vi "ExDriver.vi"(4 "Error In":errorcluster, 7 "Command":string) -> (0 "Error Out":errorcluster, 3 "Response":string)   [LabVIEW 2018]
uses:
  MOKO_LabViewLibrary/MokoLowLevel/MokoLowLovelControl/MLLC_DriverName.ctl
  MOKO_LabViewLibrary/MokoLowLevel/MokoLowLovelControl/MLLC_ConnectCluster.ctl
  MOKO_LabViewLibrary/MokoLowLevel/MokoLowLovelControl/MLLC_InterfaceType.ctl
  MOKO_LabViewLibrary/MokoLowLevel/MokoLowLovelControl/MLLC_OpenedSession.ctl
  MOKO_LabViewLibrary/MokoLowLevel/MokoLowLovelControl/MLLC_InterfaceSettings.ctl
  MOKO_LabViewLibrary/MokoLowLevel/MokoLowLovelControl/MLLC_InterfaceKind.ctl
  MOKO_LabViewLibrary/MokoLowLevel/MokoLowLovelControl/MLLC_Request.ctl
  MOKO_LabViewLibrary/MokoLowLevel/MokoLowLovelControl/MLLC_ResponseInit.ctl
panel:
  in  "Response Init":T1="43B"
  in  "Request":T2="ID"
  in  "Settings":T8={"Saved Data"=variant, "Permanent data"={"Connect"={"InterfaceType"=enum."VISA", "OpenedSession"="", "InterfaceSettings"={"Interface"=enum."RS232", "EOS 4 read"=enum."LF (\\n)", "EOS 4 write"=enum."LF (\\n)", "TMO, ms"=10000, "Sett"=variant(cluster{"Baud Rate":u32, "Data Bits":u16, "Parity":u16, "Stop Bits":u16, "Flow Control":u16, "Eho":bool} {"Baud Rate"=75, "Data Bits"=0, "Parity"=0, "Stop Bits"=0, "Flow Control"=0, "Eho"=FALSE})}}, "Values"={"Value"=0.0}}}
  in  "Error Code":u32
  in  "Driver Name":T9="ExDriver"
  in  "Mode":T10(ring)
  # "ExDriver"
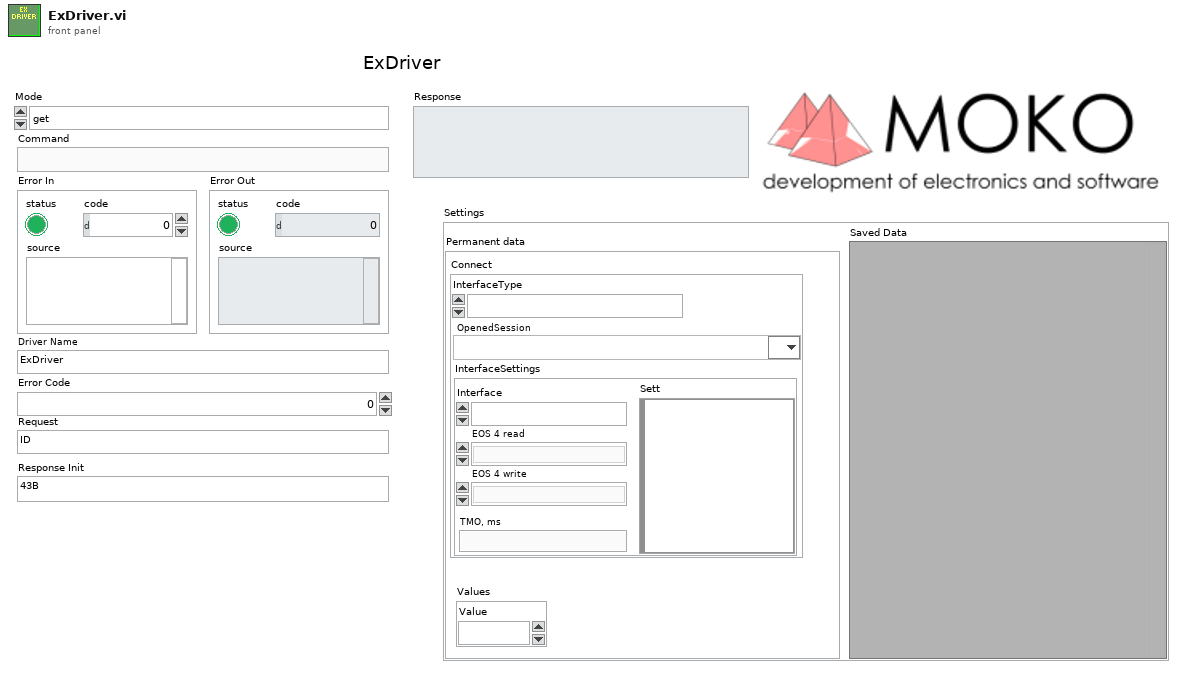
[diagram p1: front panel]
types:
  T1 = typedef "MLLC_ResponseInit.ctl" = string
  T2 = typedef "MLLC_Request.ctl" = string
  T3 = typedef "MLLC_ConnectCluster.ctl" = cluster{"InterfaceType":T4, "OpenedSession":T5, "InterfaceSettings":T6}
  T4 = typedef "MLLC_InterfaceType.ctl" = enum16{"VISA", "Prologix USB-GPIB"}
  T5 = typedef "MLLC_OpenedSession.ctl" = refnum<visa-resource-name>
  T6 = typedef "MLLC_InterfaceSettings.ctl" = cluster{"Interface":T7, "EOS 4 read":enum16{"Default (=EOS 4 write)", "CR (\\r)", "LF (\\n)", "None"}, "EOS 4 write":enum16{"CR+LF (\\r\\n)", "CR (\\r)", "LF (\\n)", "None"}, "TMO, ms":i32, "Sett":variant}
  T7 = typedef "MLLC_InterfaceKind.ctl" = enum16{"RS232", "GPIB", "USB", "Ethernet", "another"}
  T8 = cluster{"Saved Data":variant, "Permanent data":cluster{"Connect":T3, "Values":cluster{"Value":dbl}}}
  T9 = typedef "MLLC_DriverName.ctl" = string
  T10 = enum16{"get", "set", "close", "Init", "Check", "ID"}
  T11 = cluster{"Connect":T3, "Values":cluster{"Value":dbl}}
  T12 = typedef "MLLC_Mode.ctl" = enum16{"get", "set", "close", "Init", "Check"}
  T13 = typedef "MLLC_Error.ctl" = errorcluster
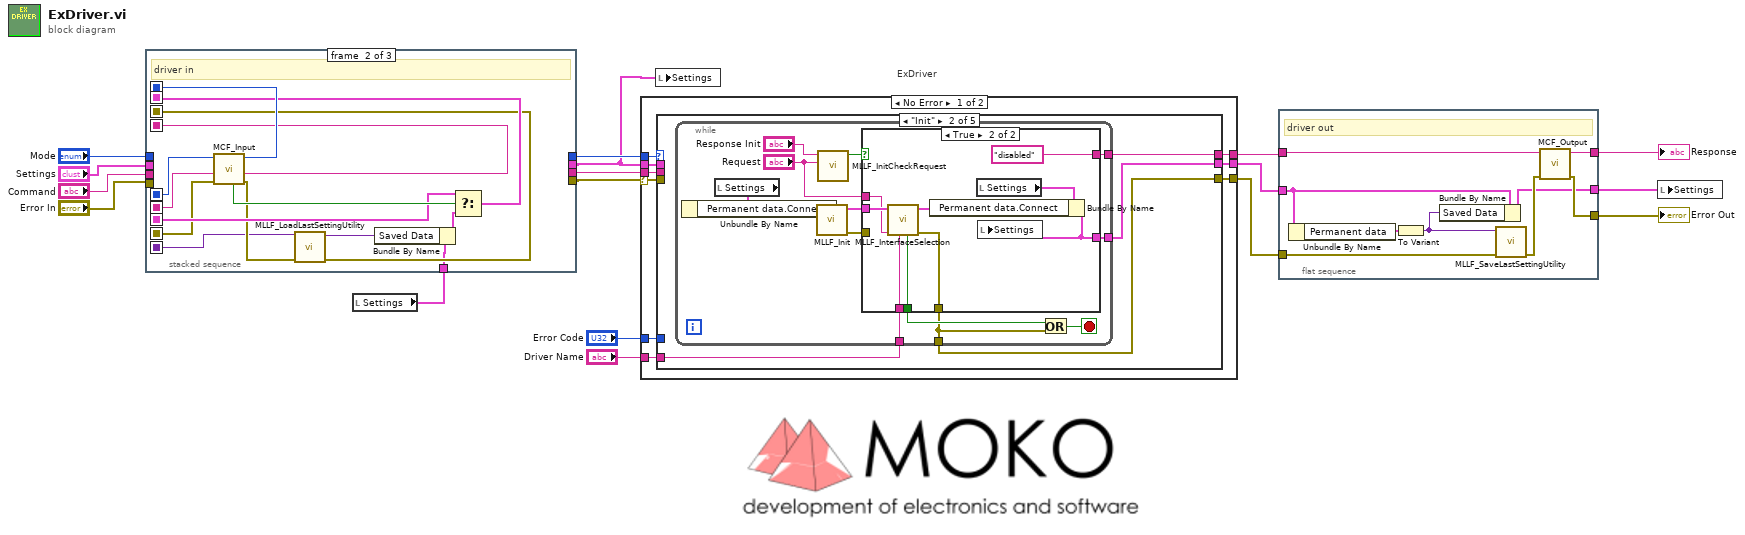
[diagram p0: block diagram]
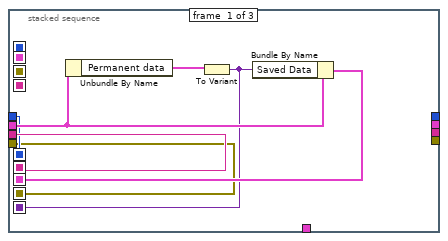
[diagram p2: hidden frame]
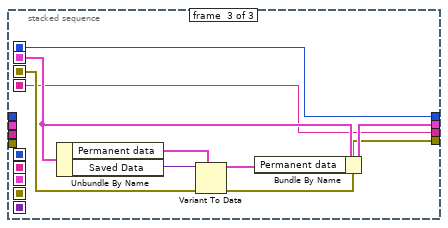
[diagram p3: hidden frame]
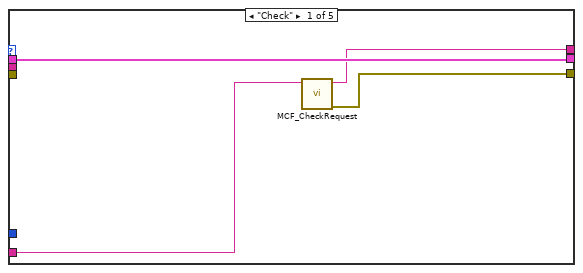
[diagram p4: hidden frame]
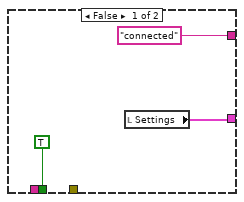
[diagram p5: hidden frame]
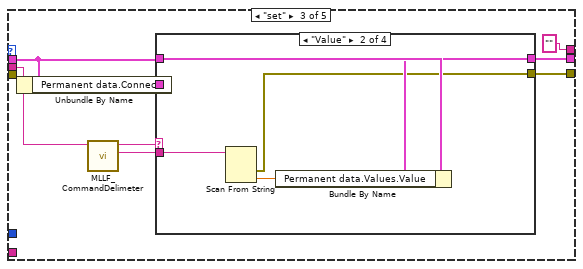
[diagram p6: hidden frame]
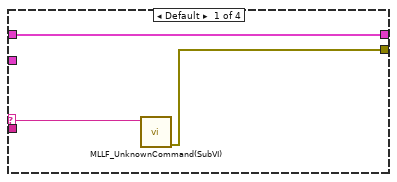
[diagram p7: hidden frame]
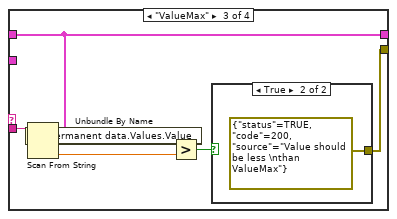
[diagram p8: hidden frame]
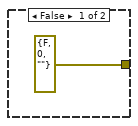
[diagram p9: hidden frame]
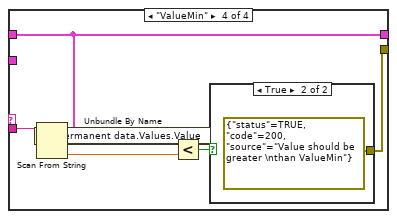
[diagram p10: hidden frame]
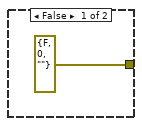
[diagram p11: hidden frame]
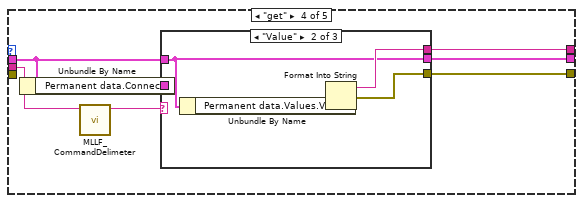
[diagram p12: hidden frame]
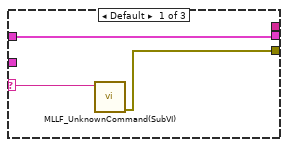
[diagram p13: hidden frame]
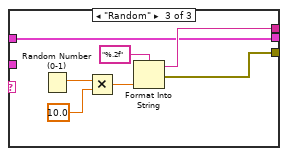
[diagram p14: hidden frame]
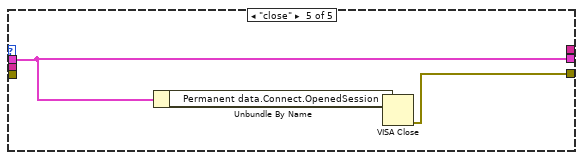
[diagram p15: hidden frame]
diagram:
  # "ExDriver"
  n1 = local read "Settings"() -> (w9:T8)
  n2 = stacked-sequence {
    seq-local: [w20 _ _] -> [_ w36 _]
    seq-local: [w19 _ _] -> [_ w37 _]
    seq-local: [w22 _ _] -> [_ w32 _]
    seq-local: [w18 _ _] -> [_ w31 _]
    seq-local: [w21 _ _] -> [_ w27 _]
    seq-local: [_ w28 _] -> [_ _ w44]
    seq-local: [_ w38 _] -> [_ _ w41]
    seq-local: [_ w35 _] -> [_ _ w40]
    seq-local: [_ w34 _] -> [_ _ w45]
    tunnel: "Command" -> [w20 _ _]
    tunnel: "Mode" -> [w19 _ _]
    tunnel: "Error In" -> [w18 _ _]
    tunnel: "Settings" -> [w23 _ _]
    tunnel: w9 -> [_ w26 _]
    tunnel: [_ _ w40] -> w5
    tunnel: [_ _ w43] -> w6
    tunnel: [_ _ w42] -> w4
    tunnel: [_ _ w41] -> w7
    frame #0 {
      n3 = Unbundle By Name(w23) -> ("Permanent data"=w24:T11)
      n4 = To Variant(anything=w24) -> (Variant=w21:variant)
      n5 = Bundle By Name(cluster=w23, "Saved Data"=w21) -> (w22:T8)
    }
    frame #1 {
      # "driver in"
      n6 = call "MCF_Input.vi"("Error In"=w31, "Command in"=w36, "Mode in"=w37) -> ("Error Out"=w30:errorcluster, "Command out"=w35:string, "Mode out"=w38:T12, "Boolean"=w33:bool)  [unwired: 5 in]
      n7 = call "MLLF_LoadLastSettingUtility.vi"("Error In"=w30, "Save data in"=w27) -> ("Error Out"=w28:errorcluster, "Save data out"=w25:variant)  [unwired: 8 in]
      n8 = Bundle By Name(cluster=w26, "Saved Data"=w25) -> (w29:T8)
      n9 = Select(t=w32, s=w33, f=w29) -> (s? t:f=w34:T8)
    }
    frame #2 {
      n10 = Unbundle By Name(w45) -> ("Permanent data"=w46:T11, "Saved Data"=w39:variant)
      n11 = Variant To Data(error in=w44, type=w46, Variant=w39) -> (data=w47:T11, error out=w42:errorcluster)
      n12 = Bundle By Name(cluster=w45, "Permanent data"=w47) -> (w43:T8)
    }
  }
  n13 = case shown="No Error" w4 {
    selector: w4 -> [w52 w147]
    tunnel: [w54 w147] -> w13
    tunnel: w7 -> [w56 _]
    tunnel: [w55 _] -> w15
    tunnel: w5 -> [w53 _]
    tunnel: w6 -> [w49 w146]
    tunnel: "Error Code" -> [w51 _]
    tunnel: "Driver Name" -> [w50 _]
    tunnel: [w48 w146] -> w14
    frame No Error {
      n14 = case shown="\"Init\"" w56 {
        tunnel: [w58 w62 "" ("Output String") w122 _] -> w55
        tunnel: [w57 w64 w90 w123 w144] -> w54
        tunnel: w53 -> [_ _ w93 w125 _]
        tunnel: w52 -> [_ _ _ _ _]
        tunnel: w51 -> [_ _ _ _ _]
        tunnel: w50 -> [w59 w61 _ _ _]
        tunnel: w49 -> [w60 _ w97 w128 w143]
        tunnel: [w60 w63 w96 w127 w143] -> w48
        frame "Check" {
          # "Проверка подленности пользователя в соответствии с протоколом MD5."
          n15 = call "MCF_CheckRequest.vi"("Driver Name"=w59) -> ("Error Out"=w57:errorcluster, "Output String"=w58:string)  [unwired: 9 in]
        }
        frame "Init" {
          # "Тут проходит инициализация оборудования"
          n16 = while {
            tunnel: [w76] -> w64
            tunnel: w61 -> [w69]
            tunnel: [w73] -> w63
            tunnel: [w70] -> w62
            stop <- w75 stop-if-true
            n17 = local read "Settings"() -> (w74:T8)
            n18 = Unbundle By Name(w74) -> ("Permanent data.Connect"=w72:T3)
            n19 = call "MLLF_Init.vi"("DriverConnect in"=w72) -> ("Error Out"=w66:errorcluster, "DriverConnect out"=w71:T3)  [unwired: 7 in]
            n20 = call "MLLF_InitCheckRequest.vi"("Answer"="Request", "Response Init"="Response Init") -> ("Design"=w67:bool)  [unwired: 6 in, 3 out]
            n21 = case shown="True" w67 {
              tunnel: w71 -> [_ w88]
              tunnel: [TRUE w84] -> w77
              tunnel: [_ w89] -> w76
              tunnel: [w79 w85] -> w73
              tunnel: ["connected" "disabled"] -> w70
              tunnel: w69 -> [_ w82]
              tunnel: w66 -> [_ _]
              tunnel: "Request" -> [_ w81]
              frame False {
                n22 = local read "Settings"() -> (w79:T8)
              }
              frame True {
                n23 = call "MLLF_InterfaceSelection.vi"("Driver Name"=w82, "Answer:"=w81, "DriverConnect in"=w88) -> ("error out"=w89:T13, "DriverConnect out"=w87:T3, "stop init?"=w84:bool)  [unwired: 4 in, 2 out]
                n24 = local read "Settings"() -> (w86:T8)
                n25 = Bundle By Name(cluster=w86, "Permanent data.Connect"=w87) -> (w85:T8)
                n26 = local write "Settings"(w85) -> ()
              }
            }
            n27 = Or(x=w77, y=w76) -> (x .or. y?=w75:bool)
          }
        }
        frame "set" {
          # "Тут реализованы функции DriverSet"
          n28 = Unbundle By Name(w97) -> ("Permanent data.Connect"=w94:T3)
          n29 = call "MLLF_CommandDelimeter.vi"("command with param"=w93) -> ("param 1"=w91:string, "command"=w92:string)  [unwired: 6 in, 3 out]
          n30 = case shown="\"Value\"" w92 {
            selector: w92 -> [w99 _ _ _]
            tunnel: [w100 w102 w106 w114] -> w96
            tunnel: w97 -> [w100 w105 w106 w114]
            tunnel: w94 -> [_ _ _ _]
            tunnel: w91 -> [_ w104 w111 w119]
            tunnel: [w98 w101 w107 w115] -> w90
            frame Default {
              n31 = call "MLLF_UnknownCommand(SubVI).vi"("Unknown command"=w99) -> ("error out"=w98:errorcluster)  [unwired: 10 in]
            }
            frame "Value" {
              n32 = Scan From String(input string=w104) -> (error out=w101:errorcluster, output 1=w103:dbl)  [unwired: 4 in, 2 out]
              n33 = Bundle By Name(cluster=w105, "Permanent data.Values.Value"=w103) -> (w102:T8)
            }
            frame "ValueMax" {
              n34 = Unbundle By Name(w106) -> ("Permanent data.Values.Value"=w109:dbl)
              n35 = Scan From String(input string=w111) -> (output 1=w110:dbl)  [unwired: 4 in, 3 out]
              n36 = Greater?(x=w109, y=w110) -> (0:w108:bool)
              n37 = case shown="True" w108 {
                tunnel: [errorcluster {"status"=FALSE, "code"=0, "source"=""} ("error IO") errorcluster {"status"=TRUE, "code"=200, "source"="Value should be less \nthan ValueMax"} ("error IO")] -> w107
                frame False {
                }
                frame True {
                }
              }
            }
            frame "ValueMin" {
              n38 = Unbundle By Name(w114) -> ("Permanent data.Values.Value"=w117:dbl)
              n39 = Scan From String(input string=w119) -> (output 1=w118:dbl)  [unwired: 4 in, 3 out]
              n40 = Less?(x=w117, y=w118) -> (x < y?=w116:bool)
              n41 = case shown="True" w116 {
                tunnel: [errorcluster {"status"=FALSE, "code"=0, "source"=""} ("error IO") errorcluster {"status"=TRUE, "code"=200, "source"="Value should be greater \nthan ValueMin"} ("error IO")] -> w115
                frame False {
                }
                frame True {
                }
              }
            }
          }
        }
        frame "get" {
          # "Тут реализованы функции DriverGet"
          n42 = Unbundle By Name(w128) -> ("Permanent data.Connect"=w126:T3)
          n43 = call "MLLF_CommandDelimeter.vi"("command with param"=w125) -> ("command"=w124:string)  [unwired: 6 in, 4 out]
          n44 = case shown="\"Value\"" w124 {
            selector: w124 -> [w130 _ _]
            tunnel: w126 -> [_ _ _]
            tunnel: w128 -> [w131 w133 w141]
            tunnel: [w131 w133 w141] -> w127
            tunnel: [w129 w132 w136] -> w123
            tunnel: [_ w134 w142] -> w122
            frame Default {
              n45 = call "MLLF_UnknownCommand(SubVI).vi"("Unknown command"=w130) -> ("error out"=w129:errorcluster)  [unwired: 10 in]
            }
            frame "Value" {
              n46 = Unbundle By Name(w133) -> ("Permanent data.Values.Value"=w135:dbl)
              n47 = Format Into String(w135) -> (resulting string=w134:string, error out=w132:errorcluster)  [unwired: 3 in]
            }
            frame "Random" {
              n48 = Random Number (0-1)() -> (number: 0 to 1=w140:dbl)
              n49 = Multiply(x=w140, y=10.0) -> (x*y=w138:dbl)
              n50 = Format Into String(format string="%.2f", w138) -> (resulting string=w142:string, error out=w136:errorcluster)  [unwired: 2 in]
            }
          }
        }
        frame "close" {
          # "Завершение сессии"
          n51 = Unbundle By Name(w143) -> ("Permanent data.Connect.OpenedSession"=w145:T5)
          n52 = VISA Close(VISA resource name=w145) -> (error out=w144:errorcluster)  [unwired: 1 in]
        }
      }
    }
    frame Error {
    }
  }
  n53 = local write "Settings"(w6) -> ()
  n54 = flat-sequence {
    tunnel: [w156] -> w11
    tunnel: [w155] -> w12
    tunnel: w15 -> [w154]
    tunnel: w13 -> [w153]
    tunnel: w14 -> [w149]
    tunnel: [w151] -> w10
    frame #0 {
      # "driver out"
      n55 = Unbundle By Name(w149) -> ("Permanent data"=w148:T11)
      n56 = To Variant(anything=w148) -> (Variant=w150:variant)
      n57 = Bundle By Name(cluster=w149, "Saved Data"=w150) -> (w151:T8)
      n58 = call "MLLF_SaveLastSettingUtility.vi"("error in"=w153, "Saved Data"=w150) -> ("error out"=w152:T13)  [unwired: 8 in, 1 out]
      n59 = call "MCF_Output.vi"("Error In"=w152, "Input"=w154) -> ("Error Out"=w155:errorcluster, "Output"=w156:string)  [unwired: 8 in]
    }
  }
  n60 = local write "Settings"(w10) -> ()
  "Response" <- w11
  "Error Out" <- w12
